vi "Sys config window-Check valid setup.vi"() -> (1 "Continue":bool)   [LabVIEW 2013]
uses:
  Typedefs/HW Setup tab control.ctl
  Globals/Sys Config window globals.vi
  <userlib>/_OpenG.lib/array/array.llb/Remove Duplicates from 1D Array (String)__ogtk.vi
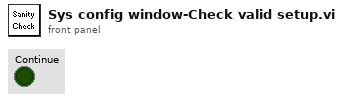
[diagram p1: front panel]
types:
  T1 = typedef "HW Setup tab control.ctl" = enum32{"Control system ", "Triggers", "DAQ FPGA", "HW Channels Setup", "XY stage", "Encoder", "System Setup", "Cameras", "AOL Properties", "Calibration Settings", "Reserved 1", "Reserved 2"}
  T2 = typedef "HW config window refs cluster.ctl" = cluster{"VI's reference":refnum<vi>, "menu reference":refnum<k9>, "Pane":refnum<vi>, "Config Tab Control":refnum<vi>, "XY stage COM port":refnum<vi>, "DAQ FPGA config cluster":refnum<vi>, "Encoder IP address":refnum<vi>, "Encoder port":refnum<vi>, "Pockels AO":refnum<vi>, "Hard shutter AO":refnum<vi>, "PMT AOs":refnum<vi>, "DO flag-Video record":refnum<vi>, "DO flag-Trial start":refnum<vi>, "Power meter AI":refnum<vi>, "XY stage available":refnum<vi>, "Encoder available":refnum<vi>, "Computer MAC address":refnum<vi>, "Externalise Triggers":refnum<vi>, "Cam VidRec available":refnum<vi>, "Triggers output setup":refnum<vi>, "AOL Properties":refnum<vi>, "Control system":T3, "Pockels cal.Zoom":refnum<vi>, "Pockels cal.Dwell time (µs)":refnum<vi>, "Laser Wavelengths ring":refnum<vi>, "AOD 5 thickness (mm)":refnum<vi>, "AOD 6 thickness (mm)":refnum<vi>, "AOD 4-5 separation (mm)":refnum<vi>, "AOD 5-6 separation (mm)":refnum<vi>, "Wheel radius (cm)":refnum<vi>, "Demo mode":refnum<vi>}
  T3 = typedef "CTRL system config cluster ref.ctl" = refnum<vi>
  T4 = typedef "CTRL system config cluster.ctl" = cluster{"Ethernet opened":bool, "Ethernet Port":u32, "Ctrl FPGA available":bool, "Ctrl FPGA Clock (MHz)":dbl, "Ctrl system MAC address":string, "Control system.Network adapter name":string, "AOD 1 Amplitude":i16, "AOD 2 Amplitude":i16, "AOD 3 Amplitude":i16, "AOD 4 Amplitude":i16, "Data Time Interval (ns)":dbl, "T0 (ns)":dbl, "Ta (ns)":dbl}
  T5 = typedef "Triggers output setup.ctl" = T6[]
  T6 = typedef "Trigger setup element cluster.ctl" = cluster{"Name":string, "Output?":bool, "Output terminal":tag, "PXI backplane line":tag, "Pulse width (us)":u16}
  T7 = typedef "DAQ FPGA config cluster.ctl" = cluster{"Ref":T8, "Target":T9, "Clock Freq (MHz) ":dbl, "input card type":T10, "Samples Wait after Trigger":u16, "AOD fill":u16, "StartupDelay":i32, "Slip Cycle (clock cycles)":u32, "Add Cycle":bool}
  T8 = typedef "FPGA Ref.ctl" = refnum<k20>
  T9 = typedef "nirio_resource_hc.ctl" = tag
  T10 = typedef "FPGA input type AC-DC.ctl" = enum16{"AC Card", "DC Card"}
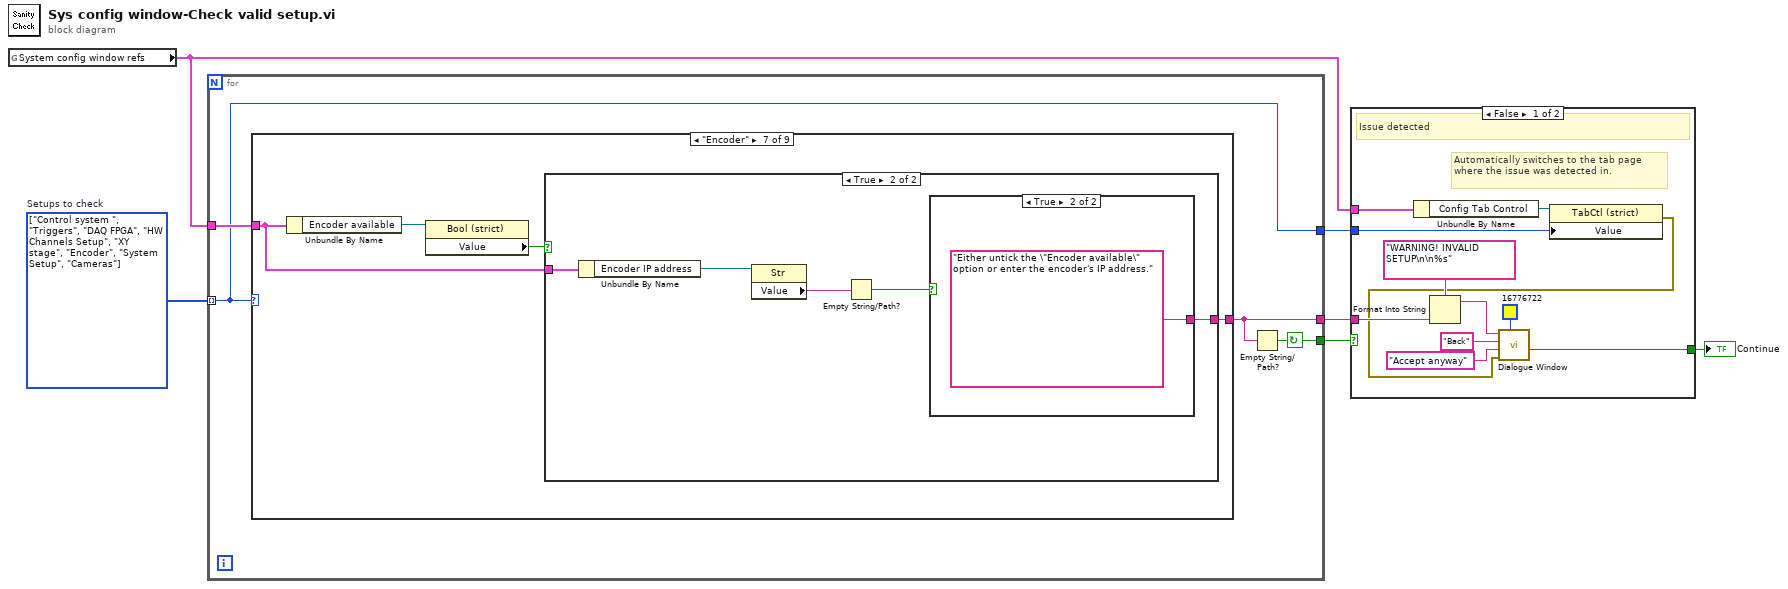
[diagram p0: block diagram]
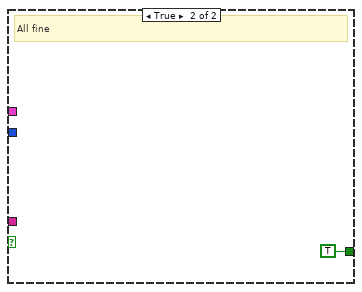
[diagram p2: hidden frame]
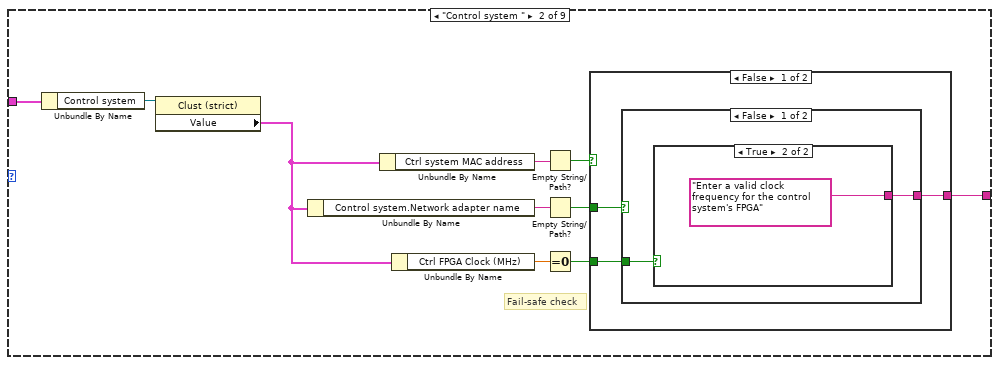
[diagram p4: hidden frame]
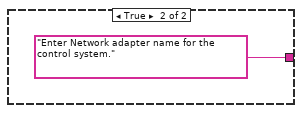
[diagram p6: hidden frame]
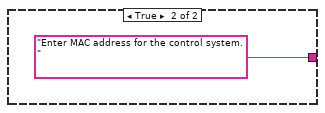
[diagram p7: hidden frame]
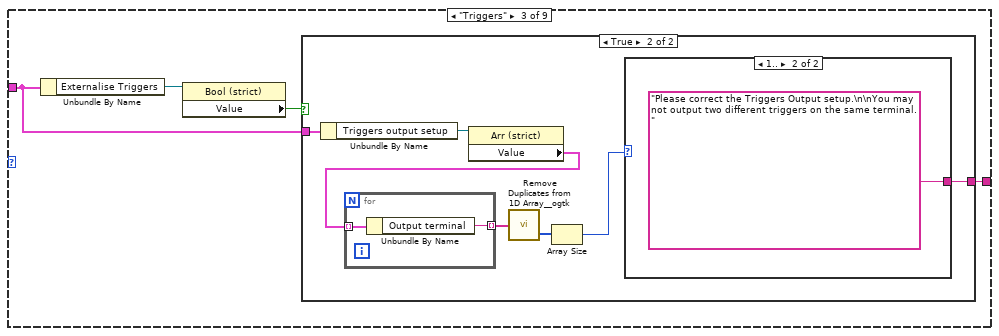
[diagram p8: hidden frame]
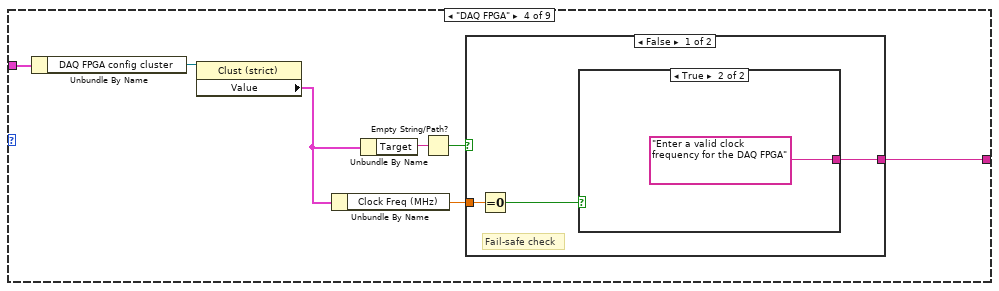
[diagram p11: hidden frame]
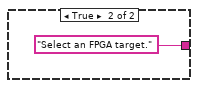
[diagram p13: hidden frame]
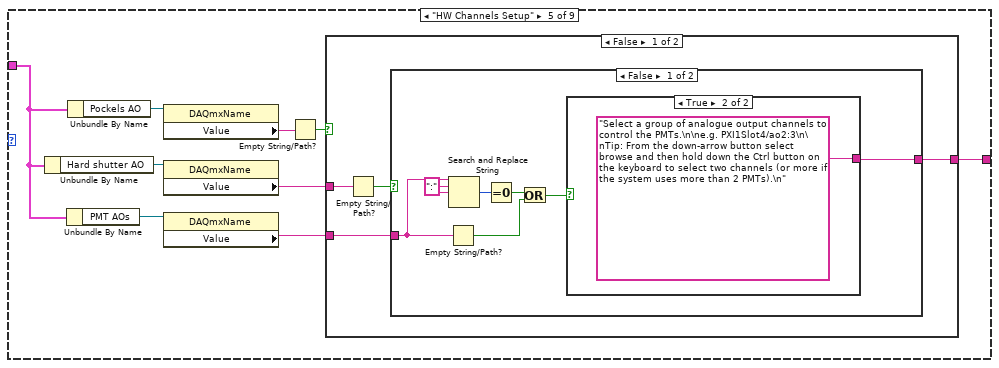
[diagram p14: hidden frame]
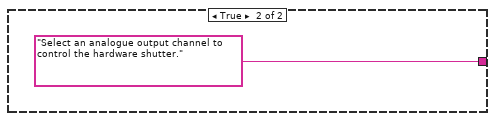
[diagram p16: hidden frame]
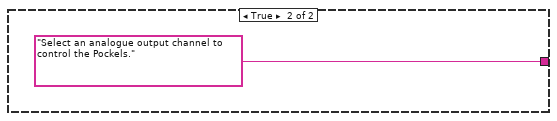
[diagram p17: hidden frame]
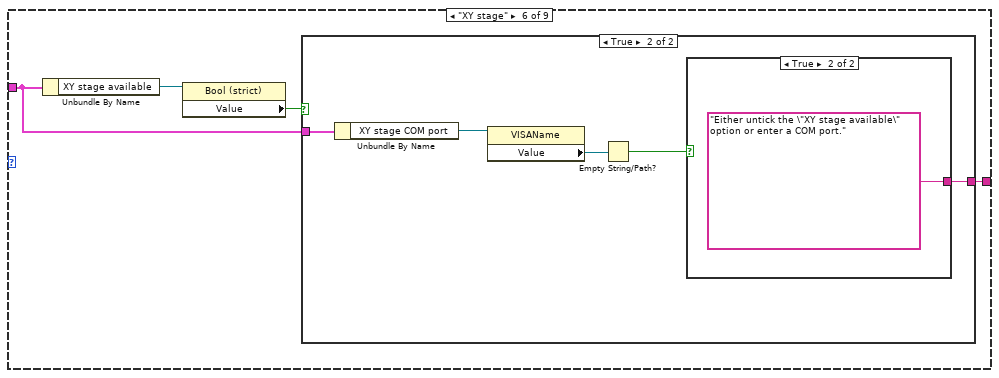
[diagram p18: hidden frame]
diagram:
  w1 = T1[] [enum."Control system ", enum."Triggers", enum."DAQ FPGA", enum."HW Channels Setup", enum."XY stage", enum."Encoder", enum."System Setup", enum."Cameras"] items=["Control system ", "Triggers", "DAQ FPGA", "HW Channels Setup", "XY stage", "Encoder", "System Setup", "Cameras", "AOL Properties", "Calibration Settings", "Reserved 1", "Reserved 2"]  # Setups to check
  n1 = global read "Sys Config window globals.vi" "System config window refs"() -> (w3:T2)
  n2 = for {
    tunnel: w3 -> [w10]
    tunnel: w1 -> [w7] mode=indexing
    tunnel: [w9] -> w5
    tunnel: [w7] -> w4
    tunnel: [w8] -> w6
    stop <- w8 continue-if-true
    n3 = case shown="\"Encoder\"" w7 {
      tunnel: w10 -> [_ w15 w32 w47 w56 w81 w91 w102 w107]
      tunnel: [_ w20 w31 w49 w60 w80 w90 w101 w106] -> w9
      frame Default {
      }
      frame "Control system " {
        # "Fail-safe check"
        n4 = Unbundle By Name(w15) -> ("Control system"=w16:T3)
        n5 = property class="Clust (strict)"(reference=w16) -> ("Value"=w14:T4)  [unwired: 1 in, 2 out]
        n6 = Unbundle By Name(w14) -> ("Control system.Network adapter name"=w12:string)
        n7 = Unbundle By Name(w14) -> ("Ctrl system MAC address"=w13:string)
        n8 = Unbundle By Name(w14) -> ("Ctrl FPGA Clock (MHz)"=w11:dbl)
        n9 = Empty String/Path?(string/path=w13) -> (empty?=w19:bool)
        n10 = Empty String/Path?(string/path=w12) -> (empty?=w18:bool)
        n11 = Equal To 0?(x=w11) -> (x = 0?=w17:bool)
        n12 = case shown="False" w19 {
          tunnel: [w23 "Enter MAC address for the control system."] -> w20
          tunnel: w18 -> [w22 _]
          tunnel: w17 -> [w21 _]
          frame False {
            n13 = case shown="False" w22 {
              tunnel: [w25 "Enter Network adapter name for the control system."] -> w23
              tunnel: w21 -> [w24 _]
              frame False {
                n14 = case shown="True" w24 {
                  tunnel: [_ "Enter a valid clock frequency for the control system's FPGA"] -> w25
                  frame False {
                  }
                  frame True {
                  }
                }
              }
              frame True {
              }
            }
          }
          frame True {
          }
        }
      }
      frame "Triggers" {
        n15 = Unbundle By Name(w32) -> ("Externalise Triggers"=w30:refnum<vi>)
        n16 = property class="Bool (strict)"(reference=w30) -> ("Value"=w29:bool)  [unwired: 1 in, 2 out]
        n17 = case shown="True" w29 {
          tunnel: w32 -> [_ w38]
          tunnel: [_ w37] -> w31
          frame False {
          }
          frame True {
            n18 = Unbundle By Name(w38) -> ("Triggers output setup"=w39:refnum<vi>)
            n19 = property class="Arr (strict)"(reference=w39) -> ("Value"=w36:T5)  [unwired: 1 in, 2 out]
            n20 = for {
              tunnel: w36 -> [w41] mode=indexing
              tunnel: [w40] -> w35 mode=indexing
              n21 = Unbundle By Name(w41) -> ("Output terminal"=w40:tag)
            }
            n22 = call-poly <userlib>:"Remove Duplicates from 1D Array__ogtk.vi"("Input Array"=w35) -> ("indices of removed elements"=w34:i32[])  [unwired: 1 out]
            n23 = Array Size(array=w34) -> (size(s)=w33:i32)
            n24 = case shown="1.." w33 {
              tunnel: [_ "Please correct the Triggers Output setup.\n\nYou may not output two different triggers on the same terminal."] -> w37
              frame 0, Default {
              }
              frame 1.. {
              }
            }
          }
        }
      }
      frame "DAQ FPGA" {
        n25 = Unbundle By Name(w47) -> ("DAQ FPGA config cluster"=w46:refnum<vi>)
        n26 = property class="Clust (strict)"(reference=w46) -> ("Value"=w45:T7)  [unwired: 1 in, 2 out]
        n27 = Unbundle By Name(w45) -> ("Clock Freq (MHz)"=w43:dbl)
        n28 = Unbundle By Name(w45) -> ("Target"=w44:T9)
        n29 = Empty String/Path?(string/path=w44) -> (empty?=w48:bool)
        n30 = case shown="False" w48 {
          tunnel: [w50 "Select an FPGA target."] -> w49
          tunnel: w43 -> [w52 _]
          frame False {
            # "Fail-safe check"
            n31 = Equal To 0?(x=w52) -> (x = 0?=w51:bool)
            n32 = case shown="True" w51 {
              tunnel: [_ "Enter a valid clock frequency for the DAQ FPGA"] -> w50
              frame False {
              }
              frame True {
              }
            }
          }
          frame True {
          }
        }
      }
      frame "HW Channels Setup" {
        n33 = Unbundle By Name(w56) -> ("Hard shutter AO"=w63:refnum<vi>)
        n34 = Unbundle By Name(w56) -> ("PMT AOs"=w57:refnum<vi>)
        n35 = Unbundle By Name(w56) -> ("Pockels AO"=w62:refnum<vi>)
        n36 = property class="DAQmxName"(reference=w62) -> ("Value"=w61:string)  [unwired: 1 in, 2 out]
        n37 = property class="DAQmxName"(reference=w63) -> ("Value"=w58:string)  [unwired: 1 in, 2 out]
        n38 = property class="DAQmxName"(reference=w57) -> ("Value"=w55:string)  [unwired: 1 in, 2 out]
        n39 = Empty String/Path?(string/path=w61) -> (empty?=w59:bool)
        n40 = case shown="False" w59 {
          tunnel: [w67 "Select an analogue output channel to control the Pockels."] -> w60
          tunnel: w58 -> [w66 _]
          tunnel: w55 -> [w64 _]
          frame False {
            n41 = Empty String/Path?(string/path=w66) -> (empty?=w65:bool)
            n42 = case shown="False" w65 {
              tunnel: [w74 "Select an analogue output channel to control the hardware shutter."] -> w67
              tunnel: w64 -> [w73 _]
              frame False {
                w72 = ":" ("search string")
                n43 = Empty String/Path?(string/path=w73) -> (empty?=w69:bool)
                n44 = Search and Replace String(input string=w73, search string=w72, replace string=w72) -> (number of replacements=w71:i32)  [unwired: 5 in, 3 out]
                n45 = Equal To 0?(x=w71) -> (x = 0?=w70:bool)
                n46 = Or(x=w70, y=w69) -> (x .or. y?=w68:bool)
                n47 = case shown="True" w68 {
                  tunnel: [_ "Select a group of analogue output channels to control the PMTs.\n\ne.g. PXI1Slot4/ao2:3\n\nTip: From the down-arrow button select browse and then hold down the Ctrl button on the keyboard to select two channels (or more if the system uses more than 2 PMTs).\n"] -> w74
                  frame False {
                  }
                  frame True {
                  }
                }
              }
              frame True {
              }
            }
          }
          frame True {
          }
        }
      }
      frame "XY stage" {
        n48 = Unbundle By Name(w81) -> ("XY stage available"=w79:refnum<vi>)
        n49 = property class="Bool (strict)"(reference=w79) -> ("Value"=w78:bool)  [unwired: 1 in, 2 out]
        n50 = case shown="True" w78 {
          tunnel: w81 -> [_ w85]
          tunnel: [_ w83] -> w80
          frame False {
          }
          frame True {
            n51 = Unbundle By Name(w85) -> ("XY stage COM port"=w86:refnum<vi>)
            n52 = property class="VISAName"(reference=w86) -> ("Value"=w84:refnum<visa-resource-name>)  [unwired: 1 in, 2 out]
            n53 = Empty String/Path?(string/path=w84) -> (empty?=w82:bool)
            n54 = case shown="True" w82 {
              tunnel: [_ "Either untick the \"XY stage available\" option or enter a COM port."] -> w83
              frame False {
              }
              frame True {
              }
            }
          }
        }
      }
      frame "Encoder" {
        n55 = Unbundle By Name(w91) -> ("Encoder available"=w89:refnum<vi>)
        n56 = property class="Bool (strict)"(reference=w89) -> ("Value"=w88:bool)  [unwired: 1 in, 2 out]
        n57 = case shown="True" w88 {
          tunnel: w91 -> [_ w95]
          tunnel: [_ w93] -> w90
          frame False {
          }
          frame True {
            n58 = Unbundle By Name(w95) -> ("Encoder IP address"=w96:refnum<vi>)
            n59 = property class="Str"(reference=w96) -> ("Value"=w94:string)  [unwired: 1 in, 2 out]
            n60 = Empty String/Path?(string/path=w94) -> (empty?=w92:bool)
            n61 = case shown="True" w92 {
              tunnel: [_ "Either untick the \"Encoder available\" option or enter the encoder's IP address."] -> w93
              frame False {
              }
              frame True {
              }
            }
          }
        }
      }
      frame "System Setup" {
        n62 = Unbundle By Name(w102) -> ("Computer MAC address"=w100:refnum<vi>)
        n63 = property class="Str"(reference=w100) -> ("Value"=w99:string)  [unwired: 1 in, 2 out]
        n64 = Empty String/Path?(string/path=w99) -> (empty?=w98:bool)
        n65 = case shown="True" w98 {
          tunnel: [_ "Enter this computer's MAC address.\nThis is required to establish connection with the control system."] -> w101
          frame False {
          }
          frame True {
          }
        }
      }
      frame "Cameras" {
        n66 = Unbundle By Name(w107) -> ("Cam VidRec available"=w105:refnum<vi>)
        n67 = property class="Bool (strict)"(reference=w105) -> ("Value"=w104:bool)  [unwired: 1 in, 2 out]
        n68 = case shown="True" w104 {
          tunnel: w107 -> [_ w114]
          tunnel: [_ w108] -> w106
          frame False {
          }
          frame True {
            n69 = Unbundle By Name(w114) -> ("DO flag-Video record"=w115:refnum<vi>)
            n70 = Unbundle By Name(w114) -> ("DO flag-Trial start"=w116:refnum<vi>)
            n71 = property class="DAQmxName"(reference=w115) -> ("Value"=w113:string)  [unwired: 1 in, 2 out]
            n72 = property class="DAQmxName"(reference=w116) -> ("Value"=w112:string)  [unwired: 1 in, 2 out]
            n73 = Empty String/Path?(string/path=w113) -> (empty?=w110:bool)
            n74 = Empty String/Path?(string/path=w112) -> (empty?=w111:bool)
            n75 = Compound Arithmetic op=OR(w110, w111) -> (w109:bool)
            n76 = case shown="True" w109 {
              tunnel: [_ "Either untick the\n\"Cameras video recording system is available\" option or specify valid digital output channels."] -> w108
              frame False {
              }
              frame True {
              }
            }
          }
        }
      }
    }
    n77 = Empty String/Path?(string/path=w9) -> (empty?=w8:bool)
  }
  n78 = case shown="False" w6 {
    tunnel: w5 -> [w124 _]
    tunnel: w4 -> [w126 _]
    tunnel: w3 -> [w128 _]
    tunnel: [w120 TRUE] -> w2
    frame False {
      # "Automatically switches to the tab page where the issue was detected in."
      # "Issue detected"
      n79 = Unbundle By Name(w128) -> ("Config Tab Control"=w127:refnum<vi>)
      n80 = Format Into String(format string="WARNING! INVALID SETUP\n\n%s" ("Message string"), w124) -> (resulting string=w123:string)  [unwired: 2 in, 1 out]
      n81 = property class="TabCtl (strict)"(reference=w127, "Value"=w126) -> (error out=w118:errorcluster)  [unwired: 1 in, 1 out]
      n82 = call "Dialogue Window.vi"("Colour"=u32 16776722, "error in (no error)"=w118, "Caption-Left button (Cancel)"="Accept anyway", "Caption-Right button (OK)"="Back", "Message string"=w123) -> ("Cancelled (Left button pressed)"=w120:bool)  [unwired: 4 in, 2 out]
    }
    frame True {
      # "All fine"
    }
  }
  "Continue" <- w2
